vi "Set configuration chain.vi"(8 "error in (no error)":errorcluster, 9 "class names":string[](array[string]), 10 "configuration":variant[](array[variant]), 11 "DAQOrcaFlash in":refnum<class "DAQOrcaFlash.lvclass">) -> (0 "error out":errorcluster, 3 "DAQOrcaFlash out":refnum<class "DAQOrcaFlash.lvclass">)   [LabVIEW 2012, in "DAQOrcaFlash.lvclass"]
uses:
  DAQOrcaFlash.lvclass
  <vilib>/Distrio/Murmex/Murmex/Murmex.lvclass
  DAQOrcaFlash.lvclass/DAQOrcaFlash.ctl
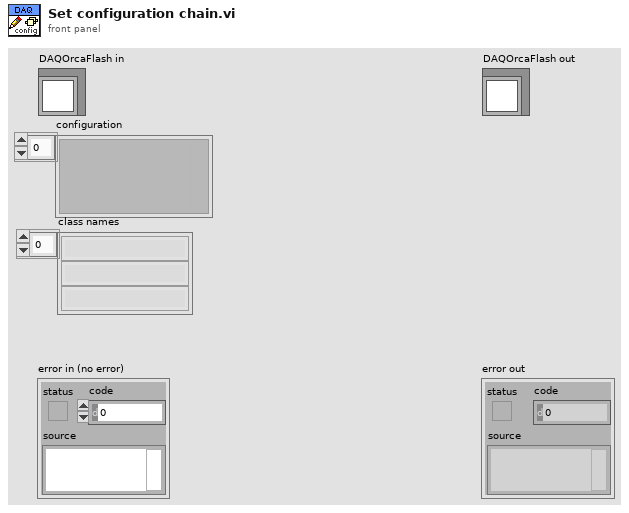
[diagram p1: front panel]
types:
  T1 = typedef "DAQOrcaFlash.lvclass/configuration_cluster.ctl" = cluster{"filepath":path, "Trigger source":T2, "Trigger mode":T3, "Sensor mode":T4, "Read out direction":T5, "Output trigger type":T6, "Output trigger source":T7, "Output trigger period":sgl[unit], "start_stop_targets":string[], "Output trigger connector":T8, "Stack component":string, "Tomo component":string, "auxiliary folders paths":path[], "maximum window size":i32, "final conversion folder":path, "Output trigger polarity":T9, "Input trigger polarity":T9, "Autofocus component":string, "enable start buttons?":bool}
  T2 = typedef "DAQOrcaFlash.lvclass/trigger_source.ctl" = sgl
  T3 = typedef "DAQOrcaFlash.lvclass/trigger_mode.ctl" = sgl
  T4 = typedef "DAQOrcaFlash.lvclass/sensor_mode.ctl" = sgl
  T5 = typedef "DAQOrcaFlash.lvclass/read out direction.ctl" = sgl
  T6 = typedef "DAQOrcaFlash.lvclass/output trigger type.ctl" = sgl
  T7 = typedef "DAQOrcaFlash.lvclass/output trigger source.ctl" = sgl
  T8 = typedef "DAQOrcaFlash.lvclass/connector.ctl" = enum32{"1", "2", "3"}
  T9 = typedef "DAQOrcaFlash.lvclass/trigger_polarity.ctl" = sgl
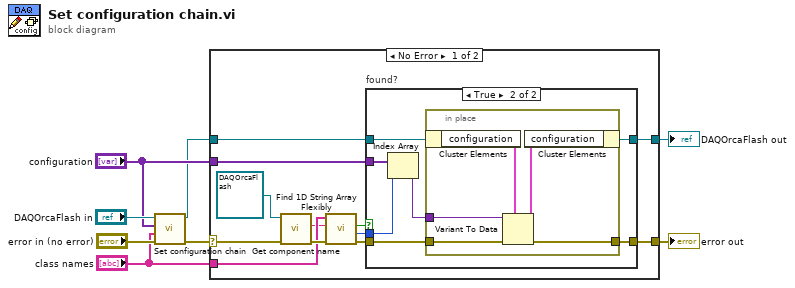
[diagram p0: block diagram]
diagram:
  n1 = call-parent "Set configuration chain.vi"("error in (no error)"="error in (no error)", "class names"="class names", "configuration"="configuration", "Murmex in"="DAQOrcaFlash in") -> ("error out"=w6:errorcluster, "Murmex out"=w4:refnum<class "DAQOrcaFlash.lvclass">)  [unwired: 6 in]
  n2 = case shown="No Error" w6 {
    selector: w6 -> [w20 w35]
    tunnel: "configuration" -> [w12 _]
    tunnel: w4 -> [w11 w36]
    tunnel: "class names" -> [w17 _]
    tunnel: [w10 w36] -> w2
    tunnel: [w9 w35] -> w1
    frame No Error {
      n3 = call <vilib>:"Get component name.vi"("error in (no error)"=w20, "Murmex in"=refnum<class "DAQOrcaFlash.lvclass"> refnum ("DAQOrcaFlash.lvclass")) -> ("error out"=w19:errorcluster, "component name"=w16:string)  [unwired: 7 in, 1 out]
      n4 = call <vilib>:"Find 1D String Array Flexibly.vi"("error in (no error)"=w19, "element"=w16, "array"=w17) -> ("error out"=w15:errorcluster, "index of element"=w14:i32, "found?"=w13:bool)  [unwired: 6 in]
      n5 = case "found?" shown="True" w13 {
        tunnel: w14 -> [_ w27]
        tunnel: w15 -> [w22 w26]
        tunnel: [w22 w25] -> w9
        tunnel: [w21 w23] -> w10
        tunnel: w11 -> [w21 w29]
        tunnel: w12 -> [_ w28]
        frame False {
        }
        frame True {
          n6 = Index Array(array=w28, index=w27) -> (element=w24:variant)
          n7 = in-place {
            in-place-border: w26 -> [w34]
            in-place-border: [w33] -> w25
            in-place-border: w24 -> [w30]
            n8 = in-place-cluster #1(w29) -> ("configuration"=w32:T1)
            n9 = Variant To Data(error in=w34, type=w32, Variant=w30) -> (data=w31:T1, error out=w33:errorcluster)
            n10 = in-place-cluster #1("configuration"=w31) -> (w23:refnum<class "DAQOrcaFlash.lvclass">)
          }
        }
      }
    }
    frame Error {
    }
  }
  "error out" <- w1
  "DAQOrcaFlash out" <- w2
